vi "ElectrodeWFM.vi"(0 "Electrode in":refnum<class "Electrode.lvclass">, 1 "Sampling Rate [Hz]":u32=100000 format="%.0p", 3 "error in (no error)":errorcluster) -> (6 "Plot On?":bool=TRUE, 7 "Electrode out":refnum<class "Electrode.lvclass">, 8 "dt [s]":dbl=0.001 format="%0.2p", 9 "Signal Array":dbl[](array[numeric]), 10 "error out":errorcluster)   [LabVIEW 2012, in "Electrode.lvclass"]
uses:
  Electrode.lvclass
  Electrode.lvclass/Electrode.ctl
  <vilib>/Analysis/NI_AALPro.lvlib
panel:
  out "Electrode Plots":waveform(dbl)[](graph)
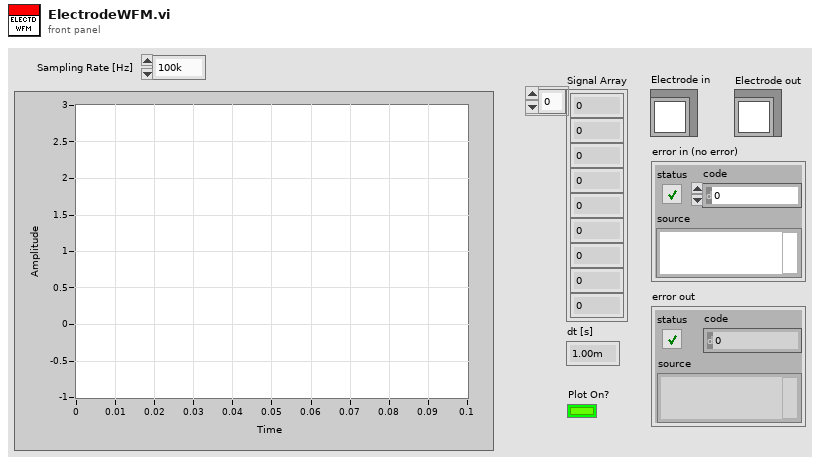
[diagram p1: front panel]
types:
  T1 = enum16{"sine", "cosine", "triangle", "square", "sawtooth", "increasing ramp", "decreasing ramp"}
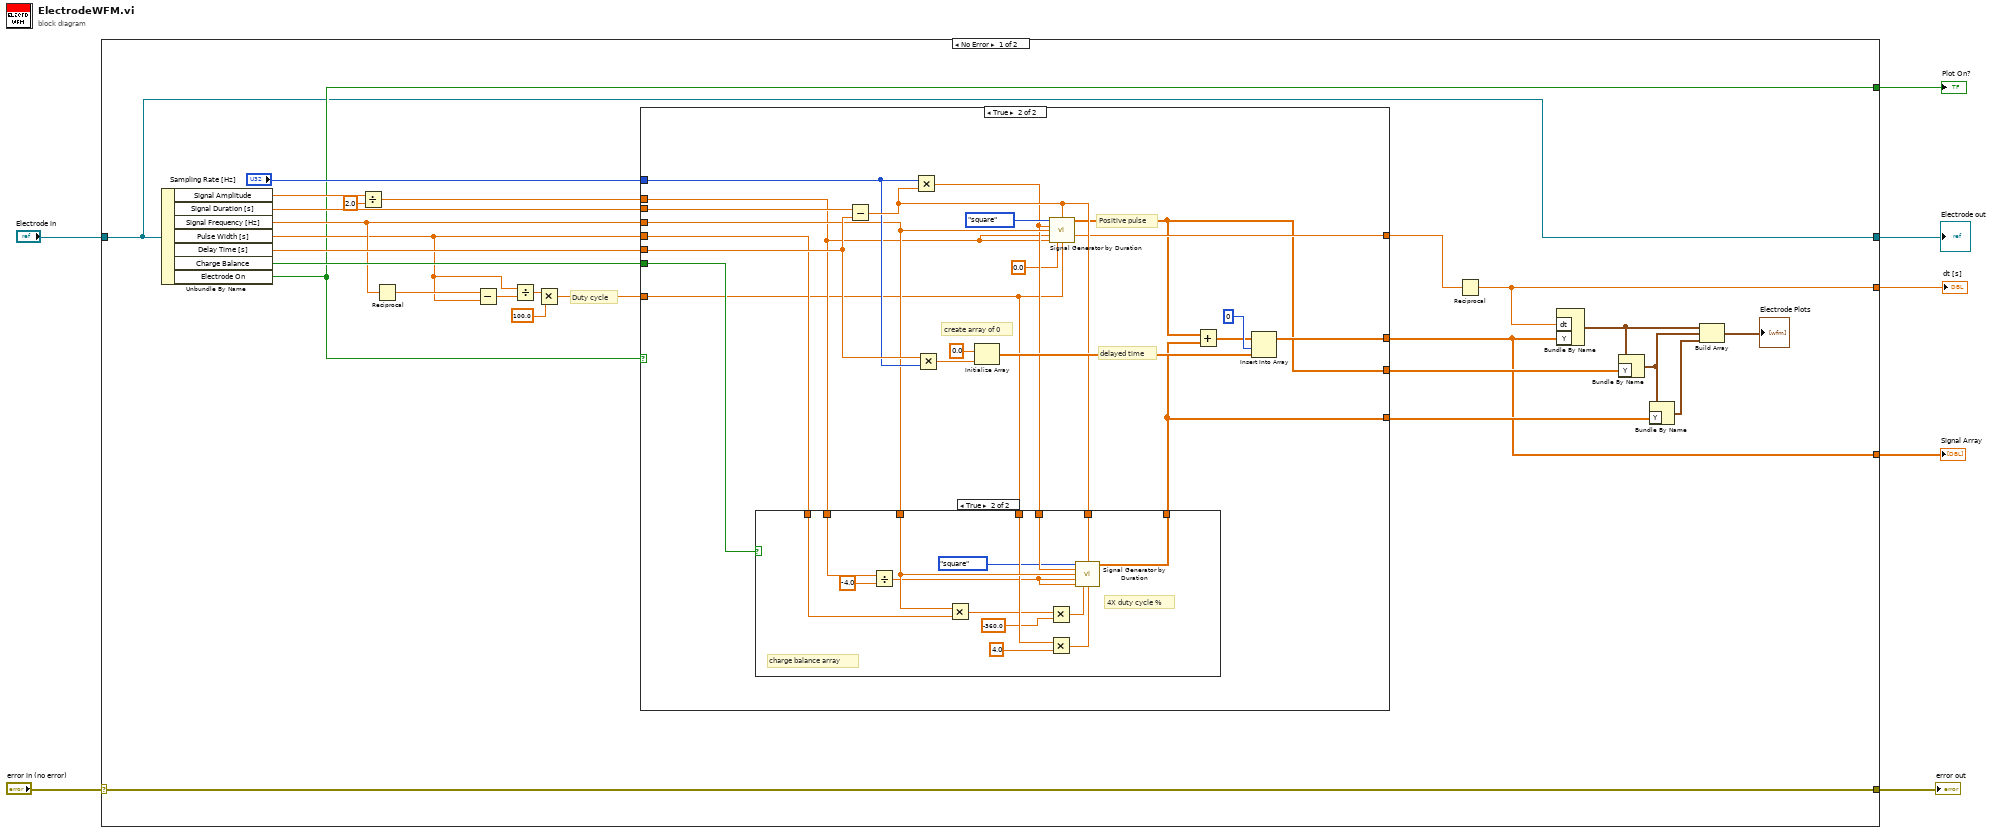
[diagram p0: block diagram]
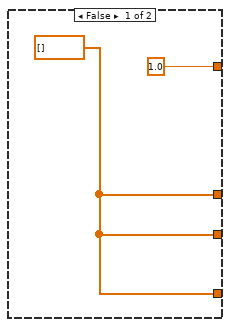
[diagram p2: hidden frame]
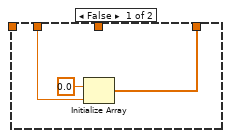
[diagram p3: hidden frame]
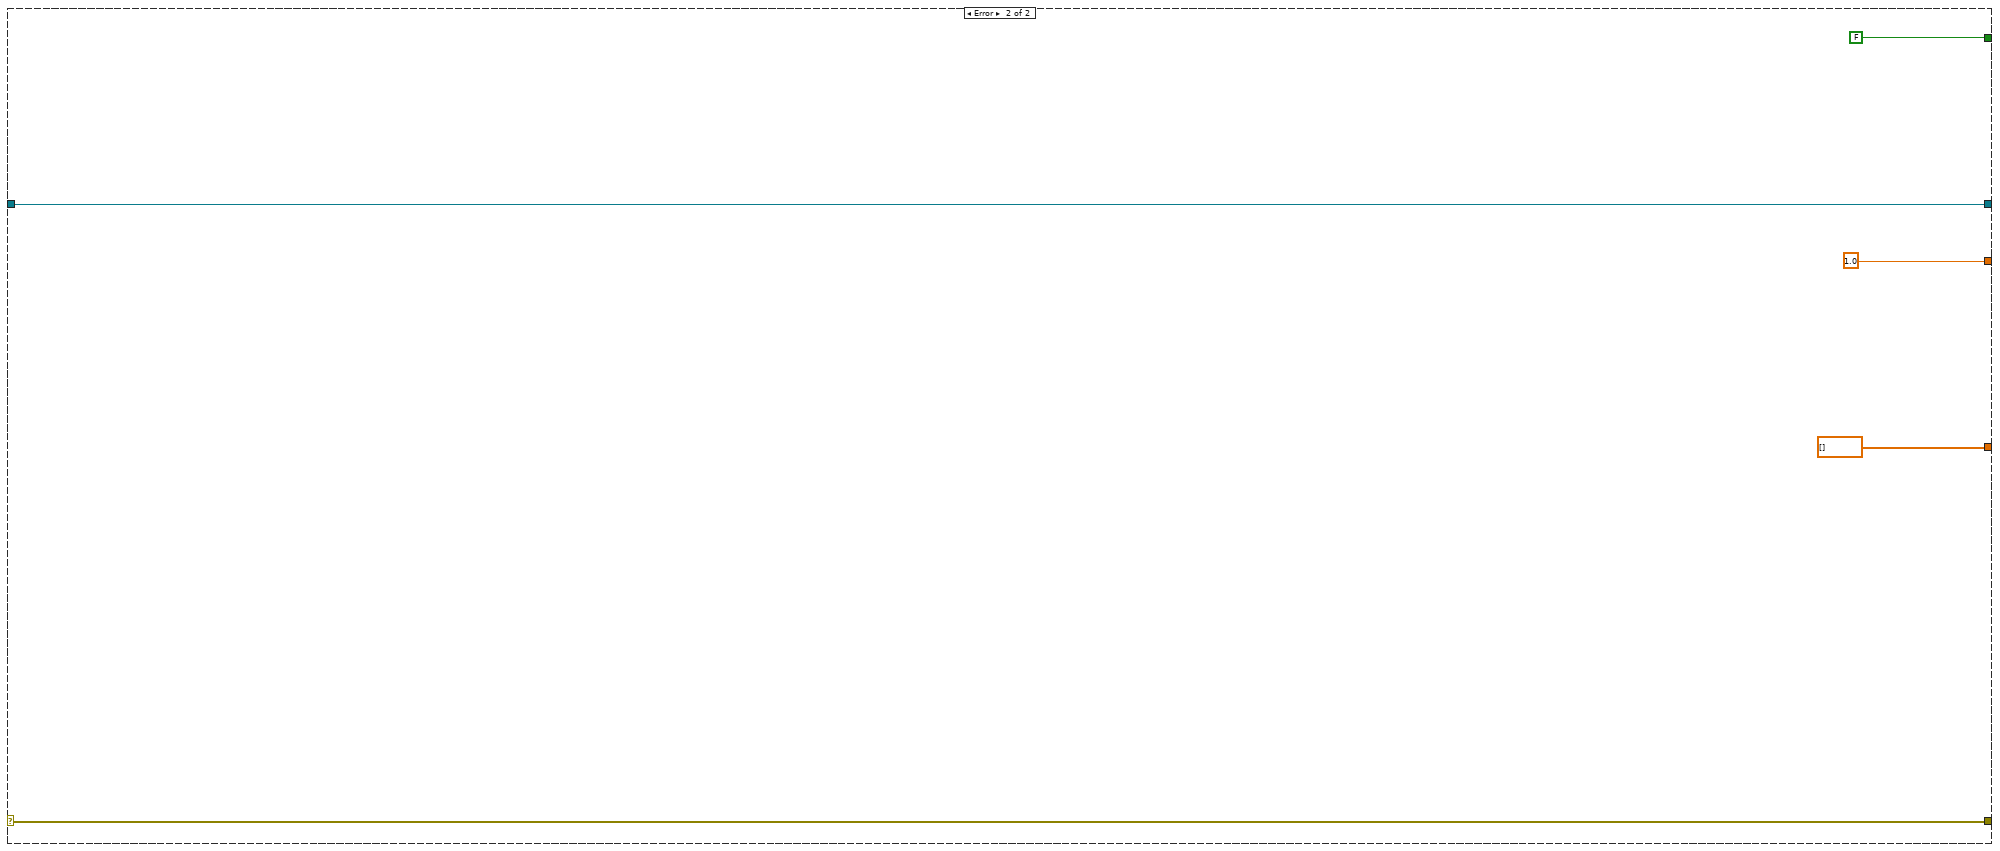
[diagram p4: hidden frame]
diagram:
  n1 = case shown="No Error" "error in (no error)" {
    selector: "error in (no error)" -> [w12 w79]
    tunnel: "Electrode in" -> [w8 w78]
    tunnel: [w12 w79] -> w5
    tunnel: [w8 w78] -> w4
    tunnel: [w11 FALSE ("Electrode On")] -> w3
    tunnel: [w10 dbl[] [] ("signal")] -> w2
    tunnel: [w9 1.0] -> w1
    frame No Error {
      # "Duty cycle"
      n2 = Unbundle By Name(w8) -> ("Signal Amplitude"=w20:dbl, "Signal Duration [s]"=w33:dbl, "Signal Frequency [Hz]"=w29:dbl, "Pulse Width [s]"=w14:dbl, "Delay Time [s]"=w32:dbl, "Charge Balance"=w31:bool, "Electrode On"=w11:bool)
      n3 = Divide(x=w20, y=2.0) -> (x/y=w19:dbl)
      n4 = Reciprocal(x=w29) -> (1/x=w15:dbl)
      n5 = Subtract(x=w15, y=w14) -> (x-y=w16:dbl)
      n6 = Divide(x=w14, y=w16) -> (x/y=w18:dbl)
      n7 = Multiply(x=w18, y=100.0) -> (x*y=w13:dbl)
      n8 = case shown="True" w11 {
        tunnel: [w34 w50] -> w10
        tunnel: "Sampling Rate [Hz]" -> [_ w45]
        tunnel: w33 -> [_ w49]
        tunnel: w29 -> [_ w43]
        tunnel: w14 -> [_ w42]
        tunnel: w32 -> [_ w48]
        tunnel: w31 -> [_ w47]
        tunnel: [1.0 ("sample rate") w44] -> w30
        tunnel: w13 -> [_ w36]
        tunnel: [w34 w41] -> w23
        tunnel: [w34 w40] -> w24
        tunnel: w19 -> [_ w37]
        frame False {
          w34 = dbl[] [] ("signal")
        }
        frame True {
          # "Positive pulse"
          # "create array of 0"
          # "delayed time"
          n9 = Subtract(x=w49, y=w48) -> (x-y=w46:dbl)
          n10 = Multiply(x=w45, y=w46) -> (x*y=w39:dbl)
          n11 = case shown="True" w47 {
            tunnel: w46 -> [_ w74]
            tunnel: w39 -> [w57 w73]
            tunnel: w37 -> [_ w72]
            tunnel: w43 -> [_ w71]
            tunnel: w36 -> [_ w70]
            tunnel: w42 -> [_ w61]
            tunnel: [w58 w62] -> w40
            frame False {
              n12 = Initialize Array(0.0 ("element"), w57) -> (w58:dbl[])
            }
            frame True {
              # "4X duty cycle %"
              # "charge balance array"
              n13 = Divide(x=w72, y=-4.0) -> (x/y=w68:dbl)
              n14 = Multiply(x=w71, y=w61) -> (x*y=w65:dbl)
              n15 = Multiply(x=w65, y=-360.0) -> (x*y=w63:dbl)
              n16 = Multiply(x=w70, y=4.0) -> (x*y=w69:dbl)
              n17 = call <vilib>:"Signal Generator by Duration.vi"("signal type"=T1."square", "duration"=w74, "# of samples"=w73, "frequency"=w71, "amplitude"=w68, "dc offset"=w68, "phase in"=w63, "square wave duty cycle (%)"=w69) -> ("signal"=w62:dbl[])  [unwired: 4 in, 3 out]
            }
          }
          n18 = Multiply(x=w48, y=w45) -> (x*y=w54:dbl)
          n19 = Initialize Array(0.0 ("amplitude"), w54) -> (w53:dbl[])
          n20 = call <vilib>:"Signal Generator by Duration.vi"("signal type"=T1."square", "duration"=w46, "# of samples"=w39, "frequency"=w43, "amplitude"=w37, "dc offset"=w37, "phase in"=0.0, "square wave duty cycle (%)"=w36) -> ("signal"=w41:dbl[], "sample rate"=w44:dbl)  [unwired: 4 in, 2 out]
          n21 = Add(x=w41, y=w40) -> (x+y=w51:dbl[])
          n22 = Insert Into Array(array=w51, index=0, new element=w53) -> (w50:dbl[])
        }
      }
      n23 = Reciprocal(x=w30) -> (1/x=w9:dbl)
      n24 = Bundle By Name("dt"=w9, "Y"=w10) -> (w27:waveform(dbl))  [unwired: 1 in]
      n25 = Bundle By Name(cluster=w27, "Y"=w23) -> (w26:waveform(dbl))
      n26 = Bundle By Name(cluster=w26, "Y"=w24) -> (w25:waveform(dbl))
      n27 = Build Array(w27, w26, w25) -> (→"Electrode Plots":waveform(dbl)[])
    }
    frame Error {
    }
  }
  "error out" <- w5
  "Electrode out" <- w4
  "Plot On?" <- w3
  "Signal Array" <- w2
  "dt [s]" <- w1
